vi "test_generic.vi"() -> ()   [LabVIEW 2010, in "GenericLightSource.lvclass"]
uses:
  GenericLightSource.lvclass
  common/classes/ErrorController/ErrorController/ErrorController.lvclass
  common/classes/XMLElement/XMLElement/XMLElement.lvclass
  common/classes/ErrorController/ErrorController/class_data.vi
  common/classes/GenericComponent/GenericComponent/GenericComponent.lvclass
panel:
  out "error loaded?":bool
  in  "adjustButton":bool
  in  "configure button":bool
  in  "stop button":bool
  in  "create OME XML button":bool
  out "OME XML":string
  in  "create button":bool
  # "Test program for LightSource components"
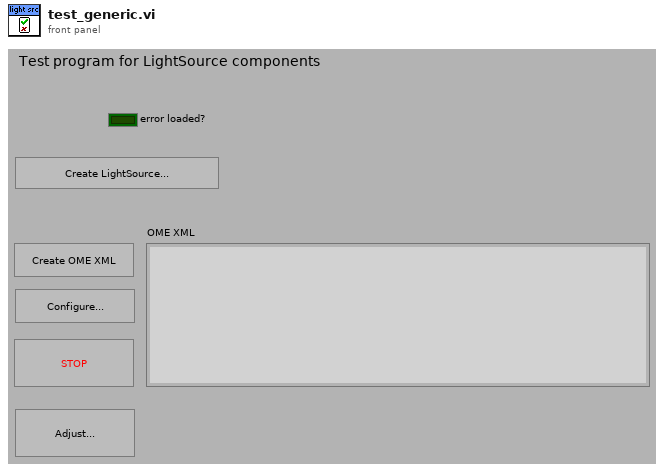
[diagram p1: front panel]
types:
  T1 = typedef "XComponentSpecification.xctl/data.ctl" = cluster{"class path":string, "configuration":string, "label":string, "settings name":string}
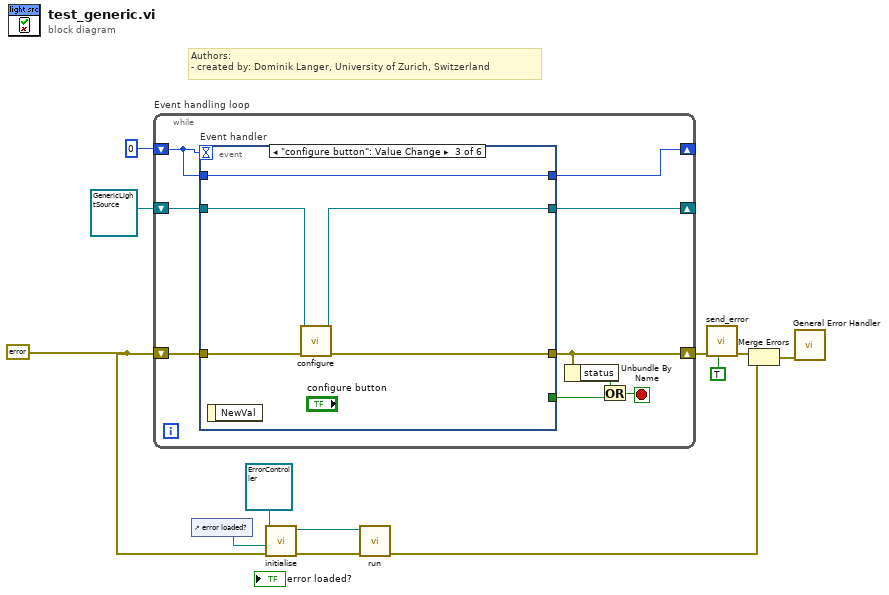
[diagram p0: block diagram]
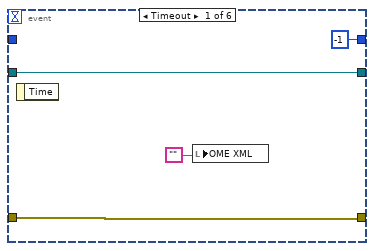
[diagram p2: hidden frame]
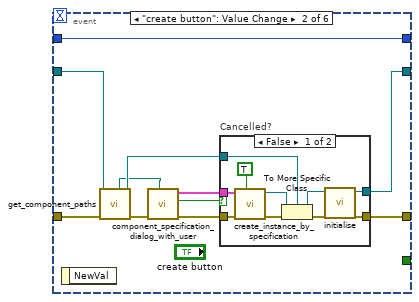
[diagram p3: hidden frame]
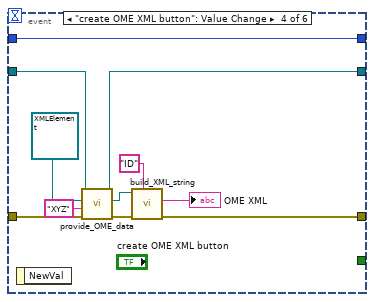
[diagram p5: hidden frame]
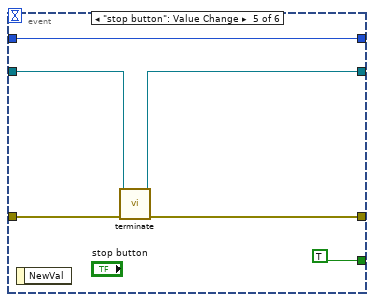
[diagram p6: hidden frame]
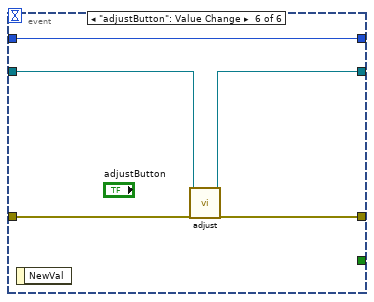
[diagram p7: hidden frame]
diagram:
  w2 = errorcluster {"status"=FALSE, "code"=0, "source"=""} ("error out")
  # "Authors: \n- created by: Dominik Langer, University of Zurich, Switzerland"
  n1 = while "Event handling loop" {
    shift-right: [w16] -> w7
    shift-left: w2 -> [w21]
    shift-right: [w19] -> _
    shift-left: 0 -> [w20]
    shift-right: [w18] -> _
    shift-left: refnum<class "GenericLightSource.lvclass"> refnum ("GenericLightSource.lvclass") -> [w17]
    stop <- w14 stop-if-true
    n2 = event "Event handler" shown="[2] \"configure button\": Value Change" {
      selector: _ -> [_ _ _ _ _ _]
      dyn-events: _ -> [_ _ _ _ _ _]
      timeout: w20 -> [_ _ _ _ _ _]
      tunnel: w21 -> [w22 w33 w52 w63 w68 w74]
      tunnel: [w22 w35 w51 w61 w67 w73] -> w16
      tunnel: [-1 w36 w53 w64 w70 w75] -> w19
      tunnel: w20 -> [_ w36 w53 w64 w70 w75]
      tunnel: [w23 w29 w49 w54 w65 w71] -> w18
      tunnel: w17 -> [w23 w31 w50 w55 w66 w72]
      tunnel: [_ _ _ _ TRUE _] -> w13
      event Timeout {
        n3 = event-data() -> ()  [unwired: 1 in, 1 out]
        n4 = local write "OME XML"("") -> ()
      }
      event "create button": Value Change {
        n5 = event-data() -> ()  [unwired: 1 in, 1 out]
        n6 = call-dynamic "get_component_paths.vi"("error in (no error)"=w33, "GenericComponent in"=w31) -> ("error out"=w34:errorcluster, "GenericComponent out"=w30:refnum<class "GenericLightSource.lvclass">, "component type directory"=w26:path)  [unwired: 4 in, 3 out]
        n7 = call "component_specification_dialog_with_user.vi"("start path"=w26, "error in (no error)"=w34) -> ("error out"=w32:errorcluster, "cancelled?"=w28:bool, "component specification out"=w27:T1)  [unwired: 7 in]
        n8 = case "Cancelled?" shown="False" w28 {
          tunnel: [w46 w47] -> w35
          tunnel: w32 -> [w40 w47]
          tunnel: w30 -> [w39 w48]
          tunnel: [w38 w48] -> w29
          tunnel: w27 -> [w37 _]
          frame False {
            n9 = call "create_instance_by_specification.vi"("call constructor?"=TRUE, "error in (no error)"=w40, "component specification"=w37) -> ("error out"=w43:errorcluster, "GenericPlugin out"=w42:refnum<class "GenericComponent.lvclass">)  [unwired: 6 in, 1 out]
            n10 = To More Specific Class(target class=w39, reference=w42, error in=w43) -> (specific class reference=w45:refnum<class "GenericLightSource.lvclass">, error out=w44:errorcluster)
            n11 = call-dynamic "initialise.vi"("error in (no error)"=w44, "GenericPlugin in"=w45) -> ("error out"=w46:errorcluster, "GenericPlugin out"=w38:refnum<class "GenericLightSource.lvclass">)  [unwired: 8 in]
          }
          frame True {
          }
        }
      }
      event "configure button": Value Change {
        n12 = event-data() -> ()  [unwired: 1 in, 1 out]
        n13 = call-dynamic "configure.vi"("error in (no error)"=w52, "GenericPlugin in"=w50) -> ("error out"=w51:errorcluster, "GenericPlugin out"=w49:refnum<class "GenericLightSource.lvclass">)  [unwired: 8 in]
      }
      event "create OME XML button": Value Change {
        n14 = event-data() -> ()  [unwired: 1 in, 1 out]
        n15 = call-dynamic "provide_OME_data.vi"("error in (no error)"=w63, "structuredAttribute string in"="XYZ" ("image ID"), "OME element in"=refnum<class "XMLElement.lvclass"> refnum ("XMLElement.lvclass"), "GenericPlugin in"=w55) -> ("error out"=w62:errorcluster, "OME element out"=w60:refnum<class "XMLElement.lvclass">, "GenericPlugin out"=w54:refnum<class "GenericLightSource.lvclass">)  [unwired: 4 in, 1 out]
        n16 = call "build_XML_string.vi"("ID tag"="ID" ("id parameter name"), "error in (no error)"=w62, "Element in"=w60) -> ("error out"=w61:errorcluster, "string"=→"OME XML":string)  [unwired: 6 in, 1 out]
      }
      event "stop button": Value Change {
        n17 = event-data() -> ()  [unwired: 1 in, 1 out]
        n18 = call-dynamic "terminate.vi"("error in (no error)"=w68, "GenericPlugin in"=w66) -> ("error out"=w67:errorcluster, "GenericPlugin out"=w65:refnum<class "GenericLightSource.lvclass">)  [unwired: 8 in]
      }
      event "adjustButton": Value Change {
        n19 = event-data() -> ()  [unwired: 1 in, 1 out]
        n20 = call-dynamic "adjust.vi"("error in (no error)"=w74, "GenericLightSource in"=w72) -> ("error out"=w73:errorcluster, "GenericLightSource out"=w71:refnum<class "GenericLightSource.lvclass">)  [unwired: 8 in]
      }
    }
    n21 = Unbundle By Name(w16) -> ("status"=w15:bool)
    n22 = Or(x=w15, y=w13) -> (x .or. y?=w14:bool)
  }
  n23 = control-ref of="error loaded?"() -> (w9:refnum<vi>)
  n24 = call-dynamic "initialise.vi"("error in (no error)"=w2, "error boolean"=w9, "ErrorController in"=refnum<class "ErrorController.lvclass"> refnum ("ErrorController.lvclass")) -> ("error out"=w11:errorcluster, "ErrorController out"=w10:refnum<class "ErrorController.lvclass">)  [unwired: 7 in]
  n25 = call "run.vi"("error in (no error)"=w11, "ErrorController in"=w10) -> ("error out"=w4:errorcluster)  [unwired: 8 in, 1 out]
  n26 = call "send_error.vi"("last error? (F)"=TRUE, "error in (no error)"=w7) -> ("error out"=w5:errorcluster)  [unwired: 9 in]
  n27 = Merge Errors(w5, w4) -> (w3:errorcluster)
  n28 = call <vilib>:"General Error Handler.vi"("error in (no error)"=w3) -> ()  [unwired: 10 in, 5 out]
